vi "set_config_cluster.vi"(8 "error in (no error)":errorcluster, 10 "config cluster variant":variant, 11 "DAQmxAnalogOut in":refnum<class "AnalogOutDL101207DAQmx.lvclass">) -> (0 "error out":errorcluster, 3 "DAQmxAnalogOut out":refnum<class "AnalogOutDL101207DAQmx.lvclass">)   [LabVIEW 2010, in "AnalogOutDL101207DAQmx.lvclass"]
uses:
  AnalogOutDL101207DAQmx.lvclass
  AnalogOutDL101207DAQmx.lvclass/AnalogOutDL101207DAQmx.ctl
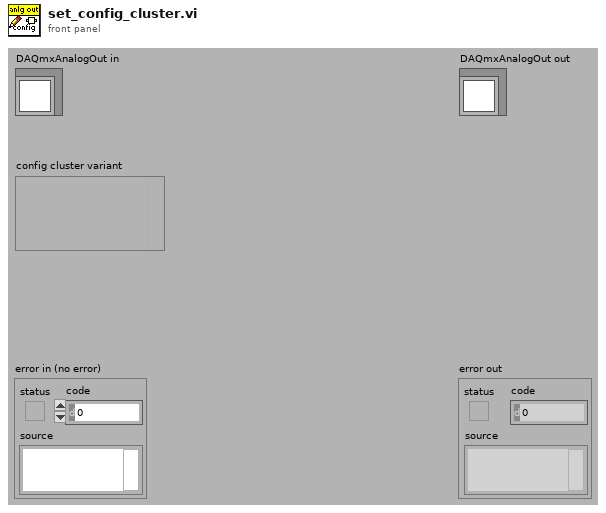
[diagram p1: front panel]
types:
  T1 = typedef "AnalogOutDL101207DAQmx.lvclass/config_data_cluster.ctl" = cluster{"physical channel":string, "minimum voltage":dbl[unit], "maximum voltage":dbl[unit], "default voltage":dbl[unit]}
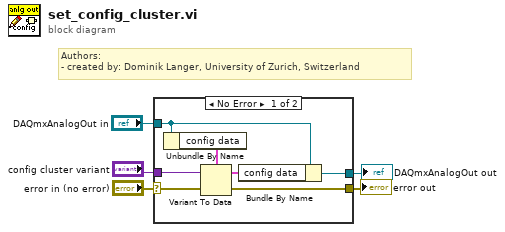
[diagram p0: block diagram]
diagram:
  # "Authors: \n- created by: Dominik Langer, University of Zurich, Switzerland"
  n1 = case shown="No Error" "error in (no error)" {
    selector: "error in (no error)" -> [w11 w13]
    tunnel: "config cluster variant" -> [w10 _]
    tunnel: "DAQmxAnalogOut in" -> [w8 w14]
    tunnel: [w7 w14] -> w2
    tunnel: [w6 w13] -> w1
    frame No Error {
      n2 = Unbundle By Name(w8) -> ("config data"=w9:T1)
      n3 = Variant To Data(error in=w11, Variant=w10, type=w9) -> (error out=w6:errorcluster, data=w12:T1)
      n4 = Bundle By Name(cluster=w8, "config data"=w12) -> (w7:refnum<class "AnalogOutDL101207DAQmx.lvclass">)
    }
    frame Error {
    }
  }
  "error out" <- w1
  "DAQmxAnalogOut out" <- w2
